vi "Sniffer.vi"() -> ()   [LabVIEW 2020, in "Serial Test.lvlib"]
uses:
  Serial Test.lvlib
  Stream-Serial/Serial Client/Serial Client.lvclass
  Sniffer Open Cmd.ctl
  lv-stream/stream/Stream/Stream.lvclass
  lv-stream/stream/Endpoint/Endpoint.lvclass
  lv-stream/stream/Connection/Connection.lvclass
  e800ee79-6252-4a27-8c84-a0a196c26224.vi
  Stream-Serial/Serial Client/Stop Bits.ctl
  Stream-Serial/Serial Client/Flow Control.ctl
  Stream-Serial/Serial Client/Parity.ctl
  Stream-Serial/Serial Client/Port Config.ctl
panel:
  out "Conn B":bool
  in  "Close":bool
  in  "Open":bool
  out "Conn A":bool
  in  "Port B":refnum<visa-resource-name>="COM6"
  in  "Port Config":T1={"Baud (115200)"=9600, "Data Bits (8)"=8, "Stop Bits (1)"=10, "Flow Control"=0, "Use LineTerm?"=FALSE, "LineTerm (\\n)"="\n", "Timeout ms (10000)"=10, "Parity (None)"=enum."None"} {"Flow Control" items=["None", "XON/XOFF", "RTS/CTS", "XON/XOFF & RTS/CTS", "DTR/DSR", "XON/XOFF & DTR/DSR"]; "Stop Bits (1)" items=["1.0"=10, "1.5"=15, "2.0"=20]}
  in  "Port A":refnum<visa-resource-name>="COM8"
  in  "Clear":bool
  out "A -> B":string
  out "A <- B":string
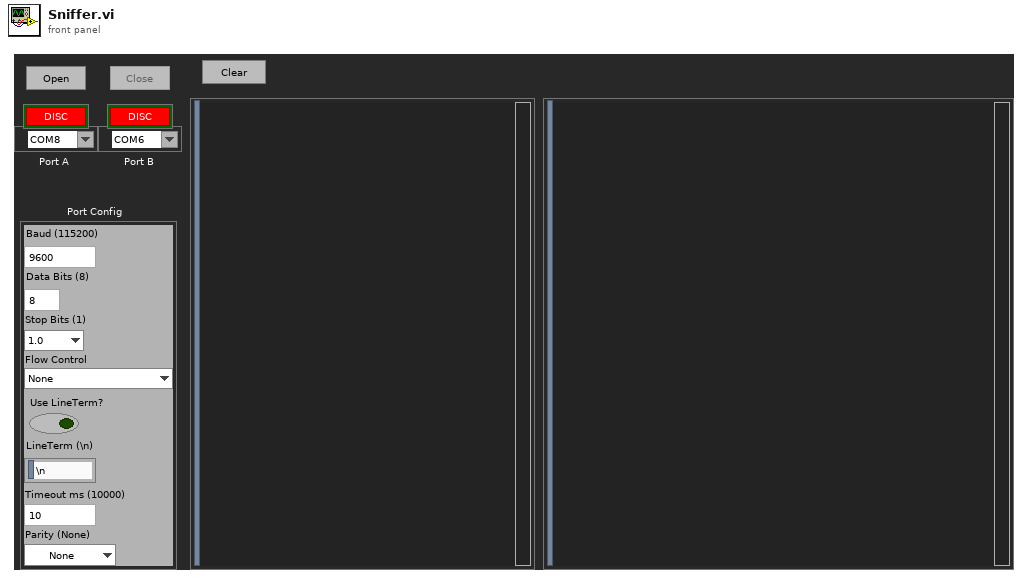
[diagram p1: front panel]
types:
  T1 = typedef "Stream-Serial.lvlib/Serial Client.lvclass/Port Config.ctl" = cluster{"Baud (115200)":u32, "Data Bits (8)":u8, "Stop Bits (1)":T2, "Flow Control":T3, "Use LineTerm?":bool, "LineTerm (\\n)":string, "Timeout ms (10000)":i32, "Parity (None)":T4}
  T2 = typedef "Stream-Serial.lvlib/Serial Client.lvclass/Stop Bits.ctl" = u16
  T3 = typedef "Stream-Serial.lvlib/Serial Client.lvclass/Flow Control.ctl" = u16
  T4 = typedef "Stream-Serial.lvlib/Serial Client.lvclass/Parity.ctl" = enum16{"None", "Odd", "Even", "Mark", "Space"}
  T5 = enum8{"Enabled", "Disabled", "Disabled and Grayed Out"}
  T6 = typedef "Serial Test.lvlib/Sniffer Open Cmd.ctl" = cluster{"Client A":refnum<class "Serial Client.lvclass">, "Client B":refnum<class "Serial Client.lvclass">}
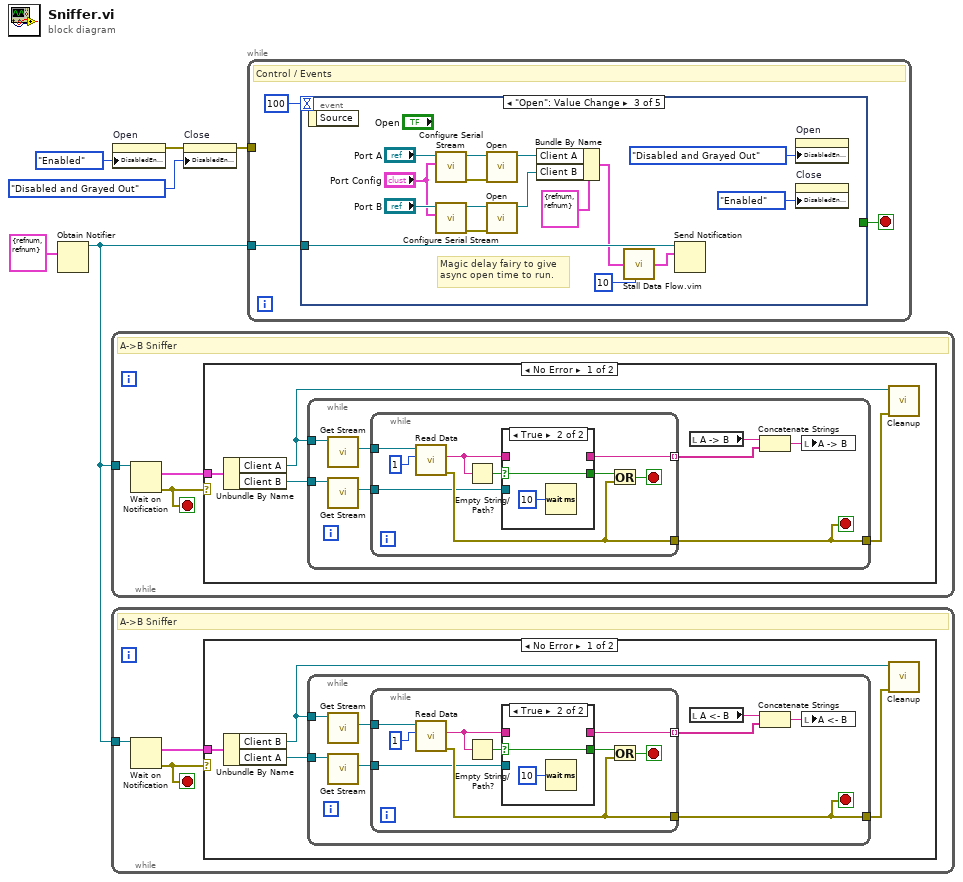
[diagram p0: block diagram]
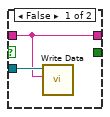
[diagram p2: hidden frame]
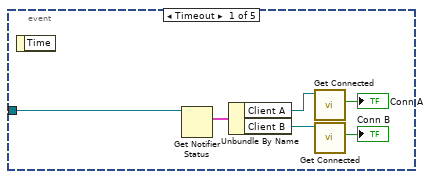
[diagram p4: hidden frame]
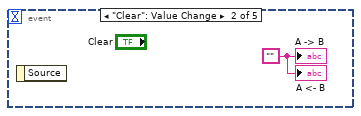
[diagram p5: hidden frame]
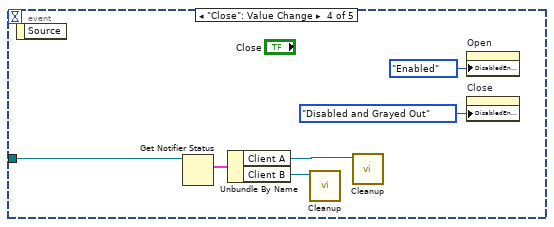
[diagram p6: hidden frame]
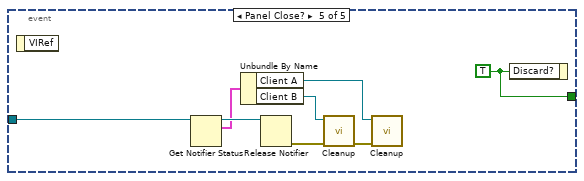
[diagram p7: hidden frame]
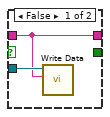
[diagram p8: hidden frame]
diagram:
  n1 = Obtain Notifier(notification data type=T6 {"Client A"=refnum, "Client B"=refnum} ("Open Cmd")) -> (notifier out=w5:refnum<notifier>)  [unwired: 3 in, 2 out]
  n2 = while {
    tunnel: w5 -> [w9]
    stop <- w7 stop-if-true
    # "A->B Sniffer"
    n3 = Wait on Notification(notifier=w9) -> (notification=w8:T6, error out=w7:errorcluster)  [unwired: 3 in, 2 out]
    n4 = case shown="No Error" w7 {
      tunnel: w8 -> [w13 _]
      frame No Error {
        n5 = Unbundle By Name(w13) -> ("Client A"=w11:refnum<class "Serial Client.lvclass">, "Client B"=w12:refnum<class "Serial Client.lvclass">)
        n6 = while {
          tunnel: w11 -> [w21]
          tunnel: w12 -> [w19]
          tunnel: [w17] -> w10
          stop <- w17 stop-if-true
          n7 = call-dynamic "Get Stream.vi"("VISA Client in"=w21) -> ("Stream"=w20:refnum<class "Stream.lvclass">)  [unwired: 8 in, 2 out]
          n8 = call-dynamic "Get Stream.vi"("VISA Client in"=w19) -> ("Stream"=w18:refnum<class "Stream.lvclass">)  [unwired: 8 in, 2 out]
          n9 = while {
            tunnel: w20 -> [w29]
            tunnel: w18 -> [w27]
            tunnel: [w30] -> w17
            tunnel: [w22] -> w15 mode=indexing
            stop <- w23 stop-if-true
            n10 = call "Read Data.vi"("Count"=1, "Stream in"=w29) -> ("error out"=w30:errorcluster, "Data"=w26:string)  [unwired: 7 in, 1 out]
            n11 = Empty String/Path?(string/path=w26) -> (empty?=w25:bool)
            n12 = case shown="True" w25 {
              selector: w25 -> [_ w34]
              tunnel: w27 -> [w32 _]
              tunnel: w26 -> [w31 _]
              tunnel: [_ w34] -> w24
              tunnel: [w31 _] -> w22
              frame False {
                n13 = call "Write Data.vi"("Data"=w31, "Stream in"=w32) -> ()  [unwired: 8 in, 2 out]
              }
              frame True {
                n14 = Wait (ms)(milliseconds to wait=u32 10) -> ()  [unwired: 1 out]
              }
            }
            n15 = Or(x=w24, y=w30) -> (x .or. y?=w23:bool)
          }
          n16 = local read "A -> B"() -> (w16:string)
          n17 = Concatenate Strings(w16, w15) -> (w14:string)
          n18 = local write "A -> B"(w14) -> ()
        }
        n19 = call-dynamic "Cleanup.vi"("error in (no error)"=w10, "VISA Client in"=w11) -> ()  [unwired: 9 in, 1 out]
      }
      frame Error {
      }
    }
  }
  n20 = while {
    tunnel: w5 -> [w37]
    stop <- w35 stop-if-true
    # "A->B Sniffer"
    n21 = Wait on Notification(notifier=w37) -> (notification=w36:T6, error out=w35:errorcluster)  [unwired: 3 in, 2 out]
    n22 = case shown="No Error" w35 {
      tunnel: w36 -> [w41 _]
      frame No Error {
        n23 = Unbundle By Name(w41) -> ("Client B"=w39:refnum<class "Serial Client.lvclass">, "Client A"=w40:refnum<class "Serial Client.lvclass">)
        n24 = while {
          tunnel: w39 -> [w49]
          tunnel: w40 -> [w47]
          tunnel: [w45] -> w38
          stop <- w45 stop-if-true
          n25 = call-dynamic "Get Stream.vi"("VISA Client in"=w49) -> ("Stream"=w48:refnum<class "Stream.lvclass">)  [unwired: 8 in, 2 out]
          n26 = call-dynamic "Get Stream.vi"("VISA Client in"=w47) -> ("Stream"=w46:refnum<class "Stream.lvclass">)  [unwired: 8 in, 2 out]
          n27 = while {
            tunnel: w48 -> [w57]
            tunnel: w46 -> [w55]
            tunnel: [w58] -> w45
            tunnel: [w50] -> w43 mode=indexing
            stop <- w51 stop-if-true
            n28 = call "Read Data.vi"("Count"=1, "Stream in"=w57) -> ("error out"=w58:errorcluster, "Data"=w54:string)  [unwired: 7 in, 1 out]
            n29 = Empty String/Path?(string/path=w54) -> (empty?=w53:bool)
            n30 = case shown="True" w53 {
              selector: w53 -> [_ w62]
              tunnel: w55 -> [w60 _]
              tunnel: w54 -> [w59 _]
              tunnel: [_ w62] -> w52
              tunnel: [w59 _] -> w50
              frame False {
                n31 = call "Write Data.vi"("Data"=w59, "Stream in"=w60) -> ()  [unwired: 8 in, 2 out]
              }
              frame True {
                n32 = Wait (ms)(milliseconds to wait=u32 10) -> ()  [unwired: 1 out]
              }
            }
            n33 = Or(x=w52, y=w58) -> (x .or. y?=w51:bool)
          }
          n34 = local read "A <- B"() -> (w44:string)
          n35 = Concatenate Strings(w44, w43) -> (w42:string)
          n36 = local write "A <- B"(w42) -> ()
        }
        n37 = call-dynamic "Cleanup.vi"("error in (no error)"=w38, "VISA Client in"=w39) -> ()  [unwired: 9 in, 1 out]
      }
      frame Error {
      }
    }
  }
  n38 = property on="Open" class="Bool"("DisabledEnum"=T5."Enabled" ("Disabled")) -> (error out=w3:errorcluster)  [unwired: 2 in, 1 out]
  n39 = property on="Close" class="Bool"(error in=w3, "DisabledEnum"=T5."Disabled and Grayed Out" ("Disabled")) -> (error out=w1:errorcluster)  [unwired: 1 in, 1 out]
  n40 = while {
    tunnel: w5 -> [w65]
    tunnel: w1 -> [_]
    stop <- w64 stop-if-true
    # "Control / Events"
    n41 = event shown="[2] \"Open\": Value Change" {
      selector: _ -> [_ _ _ _ _]
      dyn-events: _ -> [_ _ _ _ _]
      timeout: 100 -> [_ _ _ _ _]
      tunnel: w65 -> [w71 _ w79 w94 w101]
      tunnel: [_ _ _ _ w102] -> w64
      event Timeout {
        n42 = event-data() -> ()  [unwired: 1 in, 1 out]
        n43 = Get Notifier Status(notifier=w71) -> (current notification=w70:T6)  [unwired: 1 in, 4 out]
        n44 = Unbundle By Name(w70) -> ("Client A"=w68:refnum<class "Serial Client.lvclass">, "Client B"=w69:refnum<class "Serial Client.lvclass">)
        n45 = call "Get Connected.vi"("Connection in"=w68) -> ("Connected"=→"Conn A":bool)  [unwired: 8 in, 2 out]
        n46 = call "Get Connected.vi"("Connection in"=w69) -> ("Connected"=→"Conn B":bool)  [unwired: 8 in, 2 out]
      }
      event "Clear": Value Change {
        w72 = ""
        n47 = event-data() -> ()  [unwired: 1 in, 1 out]
        "A -> B" <- w72
        "A <- B" <- w72
      }
      event "Open": Value Change {
        # "Magic delay fairy to give async open time to run."
        n48 = event-data() -> ()  [unwired: 1 in, 1 out]
        n49 = call "Configure Serial Stream.vi"("Port Config (115200 8N1)"="Port Config", "Serial Port"="Port A") -> ("error out"=w84:errorcluster, "Serial Client out"=w85:refnum<class "Serial Client.lvclass">)  [unwired: 8 in]
        n50 = call "Configure Serial Stream.vi"("Port Config (115200 8N1)"="Port Config", "Serial Port"="Port B") -> ("error out"=w82:errorcluster, "Serial Client out"=w83:refnum<class "Serial Client.lvclass">)  [unwired: 8 in]
        n51 = call "Open.vi"("error in (no error)"=w84, "Endpoint in"=w85) -> ("Endpoint out"=w81:refnum<class "Serial Client.lvclass">)  [unwired: 8 in, 1 out]
        n52 = call "Open.vi"("error in (no error)"=w82, "Endpoint in"=w83) -> ("Endpoint out"=w80:refnum<class "Serial Client.lvclass">)  [unwired: 8 in, 1 out]
        n53 = Bundle By Name(cluster=T6 {"Client A"=refnum, "Client B"=refnum} ("Open Cmd"), "Client A"=w81, "Client B"=w80) -> (w75:T6)
        n54 = call "Stall Data Flow.vim"("value in"=w75, "milliseconds to wait"=u32 10) -> ("value out"=w74:T6)  [unwired: 1 out]
        n55 = Send Notification(notification=w74, notifier=w79) -> ()  [unwired: 1 in, 2 out]
        n56 = property on="Open" class="Bool"("DisabledEnum"=T5."Disabled and Grayed Out" ("Disabled")) -> ()  [unwired: 2 in, 2 out]
        n57 = property on="Close" class="Bool"("DisabledEnum"=T5."Enabled" ("Disabled")) -> ()  [unwired: 2 in, 2 out]
      }
      event "Close": Value Change {
        n58 = event-data() -> ()  [unwired: 1 in, 1 out]
        n59 = Get Notifier Status(notifier=w94) -> (current notification=w93:T6)  [unwired: 1 in, 4 out]
        n60 = Unbundle By Name(w93) -> ("Client A"=w91:refnum<class "Serial Client.lvclass">, "Client B"=w92:refnum<class "Serial Client.lvclass">)
        n61 = call-dynamic "Cleanup.vi"("VISA Client in"=w92) -> ()  [unwired: 10 in, 1 out]
        n62 = call-dynamic "Cleanup.vi"("VISA Client in"=w91) -> ()  [unwired: 10 in, 1 out]
        n63 = property on="Open" class="Bool"("DisabledEnum"=T5."Enabled" ("Disabled")) -> ()  [unwired: 2 in, 2 out]
        n64 = property on="Close" class="Bool"("DisabledEnum"=T5."Disabled and Grayed Out" ("Disabled")) -> ()  [unwired: 2 in, 2 out]
      }
      event Panel Close? {
        w102 = TRUE ("Discard?")
        n65 = event-data() -> ()  [unwired: 1 in, 1 out]
        n66 = Get Notifier Status(notifier=w101) -> (notifier out=w100:refnum<notifier>, current notification=w95:T6)  [unwired: 1 in, 3 out]
        n67 = Unbundle By Name(w95) -> ("Client A"=w98:refnum<class "Serial Client.lvclass">, "Client B"=w99:refnum<class "Serial Client.lvclass">)
        n68 = Release Notifier(notifier=w100) -> (error out=w97:errorcluster)  [unwired: 2 in, 2 out]
        n69 = call-dynamic "Cleanup.vi"("error in (no error)"=w97, "VISA Client in"=w99) -> ("error out"=w96:errorcluster)  [unwired: 9 in]
        n70 = call-dynamic "Cleanup.vi"("error in (no error)"=w96, "VISA Client in"=w98) -> ()  [unwired: 9 in, 1 out]
        n71 = event-data("Discard?"=w102) -> ()  [unwired: 1 in, 1 out]
      }
    }
  }
